vi "set plot scale V1.vi"(4 "fraction in":dbl, 7 "action":T1(ring), 8 "Coords":T3, 11 "plot scale state":T2={"Plot Ref"=refnum, "center"=0.0, "delta"=100.0, "mode"=enum."no filter", "scale cursor index"=0}) -> (0 "fraction out":dbl)   [LabVIEW 2010]
uses:
  <vilib>/Utility/miscctls.llb/LVPoint32TypeDef.ctl
  plot scale state.ctl
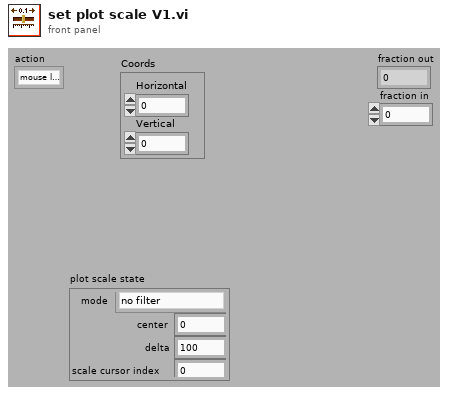
[diagram p1: front panel]
types:
  T1 = enum16{"mouse leave", "mouse enter", "mouse move", "manual zoom both", "manual zoom x", "manual zoom y"}
  T2 = typedef "plot scale state.ctl" = cluster{"Plot Ref":refnum<vi>, "center":dbl, "delta":dbl, "mode":enum16{"no filter", "median", "liner fit on median"}, "scale cursor index":i32}
  T3 = typedef "LVPoint32TypeDef.ctl" = cluster{"Horizontal":i32, "Vertical":i32}
  T4 = typedef "LVCursorListTypeDef.ctl" = cluster{"Name":string, "Color":u32, "Style":u8, "Point Style":u8, "Name Visible":bool, "Allow Drag":bool, "Cursor Mode":u32, "Plot":i32, "Index":i32, "Position":cluster{"X":dbl, "Y":dbl}, "X Scale":u32, "Y Scale":u32, "Watch Plots":i32[], "Watch All Plots":bool, "Plot Area":i32, "Label Offset":cluster{"X":dbl, "Y":dbl}}[]
  T5 = cluster{"Name":string, "Color":u32, "Style":u8, "Point Style":u8, "Name Visible":bool, "Allow Drag":bool, "Cursor Mode":u32, "Plot":i32, "Index":i32, "Position":cluster{"X":dbl, "Y":dbl}, "X Scale":u32, "Y Scale":u32, "Watch Plots":i32[], "Watch All Plots":bool, "Plot Area":i32, "Label Offset":cluster{"X":dbl, "Y":dbl}}
  T6 = typedef "LVBoundsTypeDef.ctl" = cluster{"Width":u32, "Height":u32}
  T7 = typedef "LVPositionTypeDef.ctl" = cluster{"Left":i32, "Top":i32}
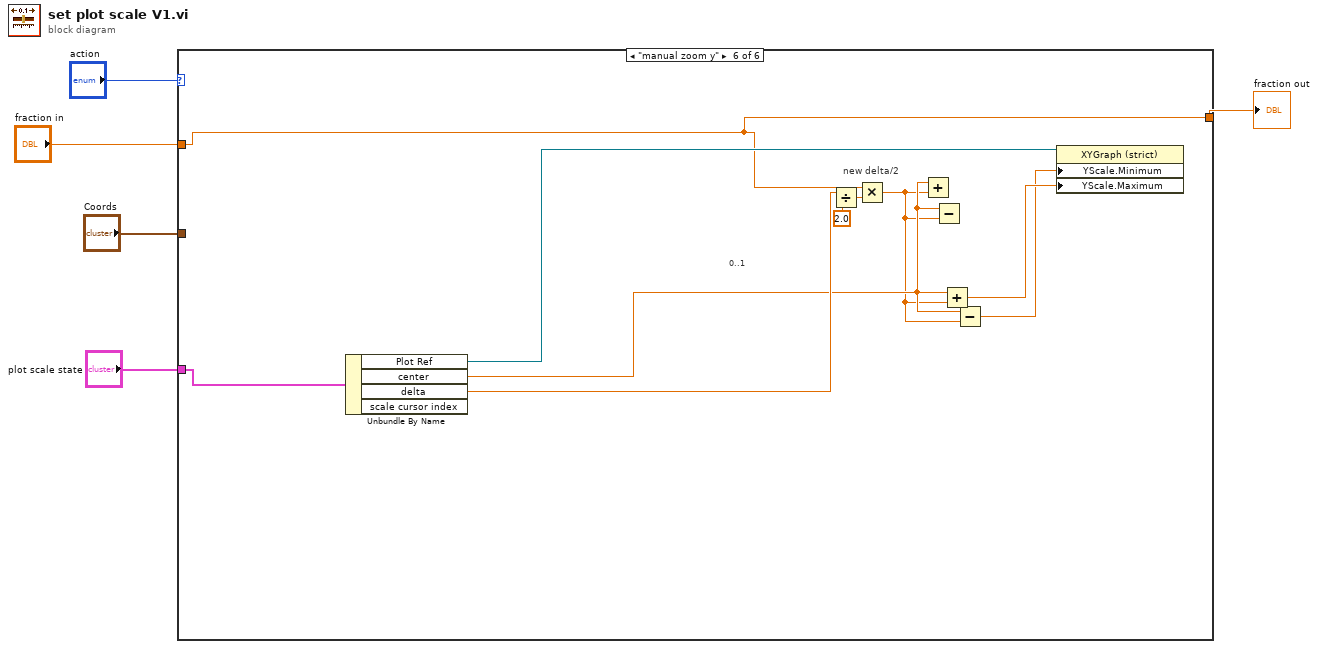
[diagram p0: block diagram]
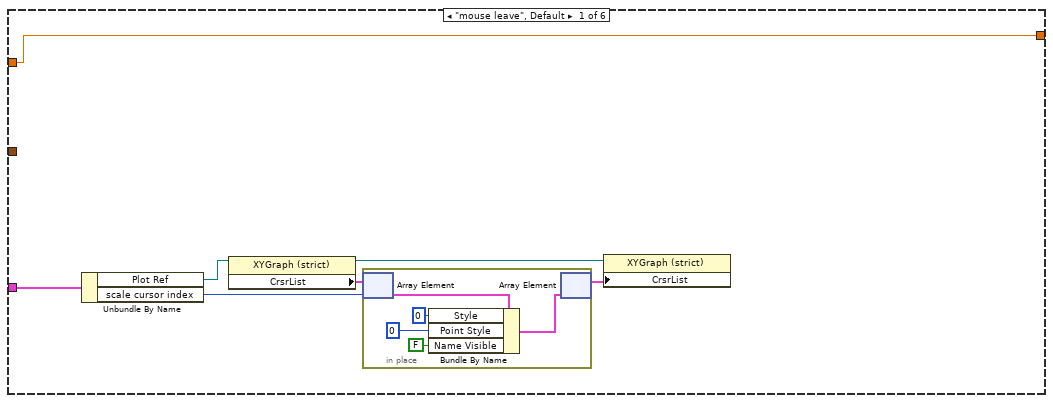
[diagram p2: hidden frame]
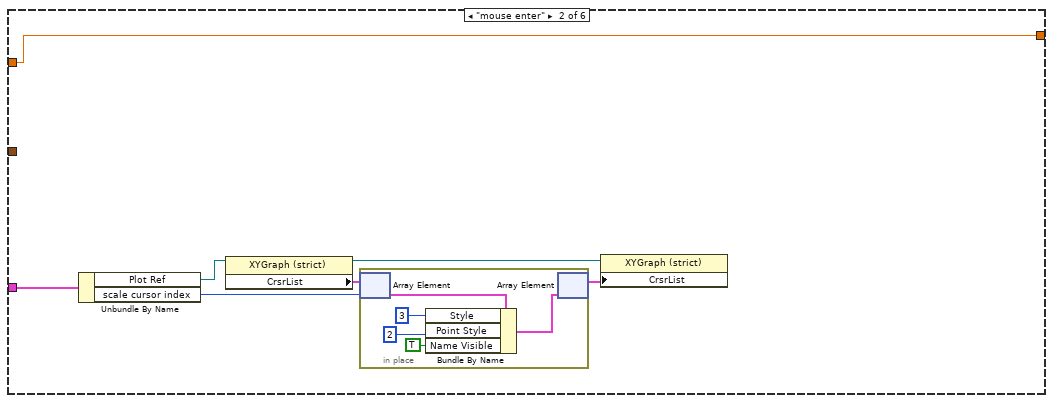
[diagram p3: hidden frame]
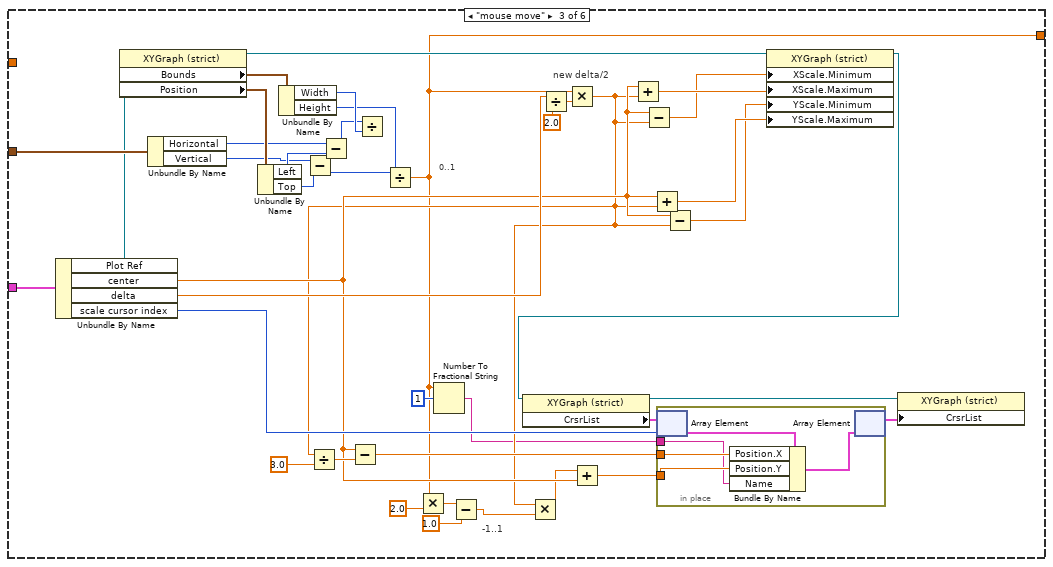
[diagram p4: hidden frame]
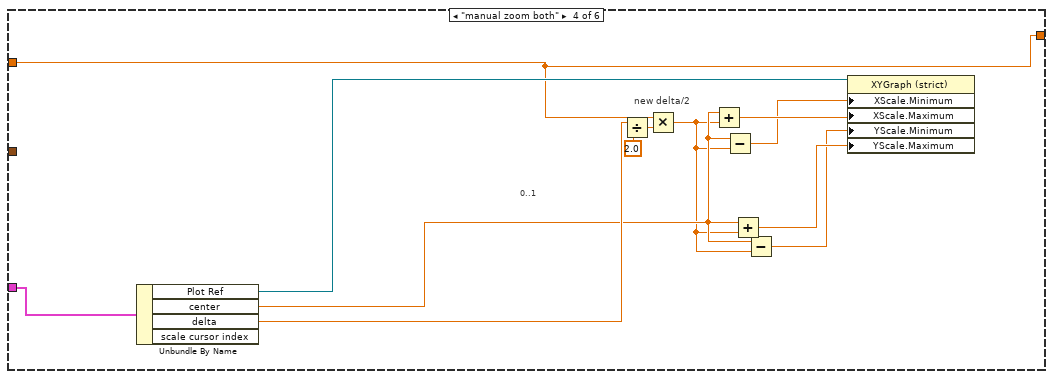
[diagram p5: hidden frame]
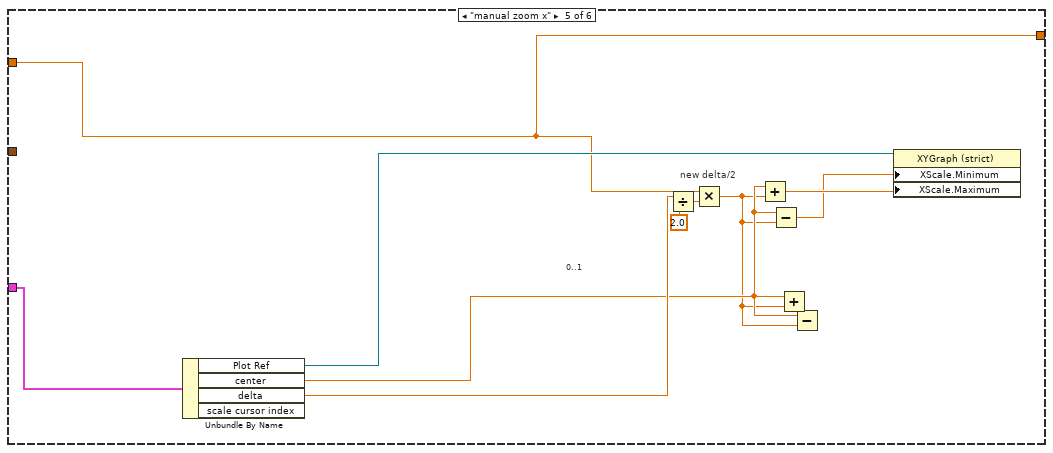
[diagram p6: hidden frame]
diagram:
  n1 = case shown="\"manual zoom y\"" "action" {
    tunnel: "Coords" -> [_ _ w52 _ _ _]
    tunnel: "plot scale state" -> [w12 w19 w46 w77 w88 w98]
    tunnel: [w6 w18 w30 w75 w87 w97] -> w2
    tunnel: "fraction in" -> [w6 w18 _ w75 w87 w97]
    frame "mouse leave", Default {
      n2 = Unbundle By Name(w12) -> ("Plot Ref"=w11:refnum<vi>, "scale cursor index"=w9:i32)
      n3 = property on="Property Node" class="XYGraph (strict)"(reference=w11) -> (reference out=w7:refnum<vi>, "CrsrList"=w10:T4)  [unwired: 1 in, 1 out]
      n4 = in-place {
        n5 = in-place-array #1(w10, w9) -> (w17:T5)
        n6 = Bundle By Name(cluster=w17, "Style"=u8 0, "Point Style"=u8 0, "Name Visible"=FALSE) -> (w16:T5)
        n7 = in-place-array #1(w16) -> (w8:T4)  [unwired: 1 out]
      }
      n8 = property on="Property Node" class="XYGraph (strict)"(reference=w7, "CrsrList"=w8) -> ()  [unwired: 1 in, 2 out]
    }
    frame "mouse enter" {
      n9 = Unbundle By Name(w19) -> ("Plot Ref"=w24:refnum<vi>, "scale cursor index"=w22:i32)
      n10 = property on="Property Node" class="XYGraph (strict)"(reference=w24) -> (reference out=w20:refnum<vi>, "CrsrList"=w23:T4)  [unwired: 1 in, 1 out]
      n11 = in-place {
        n12 = in-place-array #2(w23, w22) -> (w29:T5)
        n13 = Bundle By Name(cluster=w29, "Style"=u8 3, "Point Style"=u8 2, "Name Visible"=TRUE) -> (w28:T5)
        n14 = in-place-array #2(w28) -> (w21:T4)  [unwired: 1 out]
      }
      n15 = property on="Property Node" class="XYGraph (strict)"(reference=w20, "CrsrList"=w21) -> ()  [unwired: 1 in, 2 out]
    }
    frame "mouse move" {
      # "-1..1"
      # "0..1"
      # "new delta/2"
      n16 = Unbundle By Name(w46) -> ("Plot Ref"=w50:refnum<vi>, "center"=w38:dbl, "delta"=w51:dbl, "scale cursor index"=w45:i32)
      n17 = property on="Property Node" class="XYGraph (strict)"(reference=w50) -> (reference out=w64:refnum<vi>, "Bounds"=w63:T6, "Position"=w69:T7)  [unwired: 1 in, 1 out]
      n18 = Unbundle By Name(w52) -> ("Horizontal"=w68:i32, "Vertical"=w66:i32)
      n19 = Unbundle By Name(w69) -> ("Left"=w67:i32, "Top"=w65:i32)
      n20 = Unbundle By Name(w63) -> ("Width"=w62:u32, "Height"=w61:u32)
      n21 = Subtract(x=w66, y=w65) -> (x-y=w53:i32)
      n22 = Subtract(x=w68, y=w67) -> (x-y=w54:i32)
      n23 = Divide(x=w54, y=w62) -> ()  [unwired: 1 out]
      n24 = Divide(x=w53, y=w61) -> (x/y=w30:dbl)
      n25 = Multiply(x=w30, y=2.0) -> (x*y=w40:dbl)
      n26 = Number To Fractional String(number=w30, width (-)=i16 1) -> (F-format string=w31:string)  [unwired: 2 in]
      n27 = Subtract(x=w40, y=1.0) -> (x-y=w33:dbl)
      n28 = Divide(x=w51, y=2.0) -> (x/y=w59:dbl)
      n29 = Multiply(x=w30, y=w59) -> (x*y=w35:dbl)
      n30 = Divide(x=w35, y=3.0) -> (x/y=w42:dbl)
      n31 = Subtract(x=w38, y=w42) -> (x-y=w41:dbl)
      n32 = Multiply(x=w35, y=w33) -> (x*y=w37:dbl)
      n33 = Add(x=w37, y=w38) -> (x+y=w36:dbl)
      n34 = Add(x=w38, y=w35) -> (x+y=w58:dbl)
      n35 = Subtract(x=w38, y=w35) -> (x-y=w57:dbl)
      n36 = Add(x=w38, y=w35) -> (x+y=w56:dbl)
      n37 = Subtract(x=w38, y=w35) -> (x-y=w55:dbl)
      n38 = property on="Property Node" class="XYGraph (strict)"(reference=w64, "XScale.Minimum"=w57, "XScale.Maximum"=w58, "YScale.Minimum"=w55, "YScale.Maximum"=w56) -> (reference out=w44:refnum<vi>)  [unwired: 1 in, 1 out]
      n39 = property on="Property Node" class="XYGraph (strict)"(reference=w44) -> (reference out=w47:refnum<vi>, "CrsrList"=w49:T4)  [unwired: 1 in, 1 out]
      n40 = in-place {
        in-place-border: w41 -> [w72]
        in-place-border: w36 -> [w71]
        in-place-border: w31 -> [w70]
        n41 = in-place-array #3(w49, w45) -> (w74:T5)
        n42 = Bundle By Name(cluster=w74, "Position.X"=w72, "Position.Y"=w71, "Name"=w70) -> (w73:T5)
        n43 = in-place-array #3(w73) -> (w48:T4)  [unwired: 1 out]
      }
      n44 = property on="Property Node" class="XYGraph (strict)"(reference=w47, "CrsrList"=w48) -> ()  [unwired: 1 in, 2 out]
    }
    frame "manual zoom both" {
      # "0..1"
      # "new delta/2"
      n45 = Unbundle By Name(w77) -> ("Plot Ref"=w76:refnum<vi>, "center"=w79:dbl, "delta"=w80:dbl)  [unwired: 1 out]
      n46 = Divide(x=w80, y=2.0) -> (x/y=w85:dbl)
      n47 = Multiply(x=w75, y=w85) -> (x*y=w78:dbl)
      n48 = Add(x=w79, y=w78) -> (x+y=w84:dbl)
      n49 = Subtract(x=w79, y=w78) -> (x-y=w83:dbl)
      n50 = Add(x=w79, y=w78) -> (x+y=w82:dbl)
      n51 = Subtract(x=w79, y=w78) -> (x-y=w81:dbl)
      n52 = property on="Property Node" class="XYGraph (strict)"(reference=w76, "XScale.Minimum"=w83, "XScale.Maximum"=w84, "YScale.Minimum"=w81, "YScale.Maximum"=w82) -> ()  [unwired: 1 in, 2 out]
    }
    frame "manual zoom x" {
      # "0..1"
      # "new delta/2"
      n53 = Unbundle By Name(w88) -> ("Plot Ref"=w89:refnum<vi>, "center"=w91:dbl, "delta"=w92:dbl)  [unwired: 1 out]
      n54 = Divide(x=w92, y=2.0) -> (x/y=w95:dbl)
      n55 = Multiply(x=w87, y=w95) -> (x*y=w90:dbl)
      n56 = Add(x=w91, y=w90) -> (x+y=w94:dbl)
      n57 = Subtract(x=w91, y=w90) -> (x-y=w93:dbl)
      n58 = Add(x=w91, y=w90) -> ()  [unwired: 1 out]
      n59 = Subtract(x=w91, y=w90) -> ()  [unwired: 1 out]
      n60 = property on="Property Node" class="XYGraph (strict)"(reference=w89, "XScale.Minimum"=w93, "XScale.Maximum"=w94) -> ()  [unwired: 1 in, 2 out]
    }
    frame "manual zoom y" {
      # "0..1"
      # "new delta/2"
      n61 = Unbundle By Name(w98) -> ("Plot Ref"=w99:refnum<vi>, "center"=w101:dbl, "delta"=w102:dbl)  [unwired: 1 out]
      n62 = Divide(x=w102, y=2.0) -> (x/y=w105:dbl)
      n63 = Multiply(x=w97, y=w105) -> (x*y=w100:dbl)
      n64 = Add(x=w101, y=w100) -> ()  [unwired: 1 out]
      n65 = Subtract(x=w101, y=w100) -> ()  [unwired: 1 out]
      n66 = Add(x=w101, y=w100) -> (x+y=w104:dbl)
      n67 = Subtract(x=w101, y=w100) -> (x-y=w103:dbl)
      n68 = property on="Property Node" class="XYGraph (strict)"(reference=w99, "YScale.Minimum"=w103, "YScale.Maximum"=w104) -> ()  [unwired: 1 in, 2 out]
    }
  }
  "fraction out" <- w2
